vi "coag model selector.vi"(10 "scans":i32, 11 "Coagulant":T2={"flocculator volume (L)"=100.0, "clarifier volume (L)"=0.0, "dose updates per HRT"=0, "target clarified turbidity (NTU)"=0.3, "Coagulant mode"=enum."manual", "Coag dose [mg/L]"=0.0, "pump mL/rev"=0.0, "clarifier flow [L/s]"=0.5, "min Coag dose [mg/L]"=0.0, "max Coag dose [mg/L]"=0.0, "Steps"=3, "HRT response delay"=1, "Ku*"=1.0} {"HRT response delay" min=1 max=10 step=1; "Steps" min=3 step=1; "clarifier flow [L/s]" min=0.0001 max=1.0 step=0.0001; "target clarified turbidity (NTU)" min=0.1 max=5.0 step=0.01; "dose updates per HRT" min=1 max=100 step=1}) -> (7 "coag model":T1)   [LabVIEW 2019]
uses:
  coag.ctl
  model type.ctl
panel:
  # "min"
  # "max"
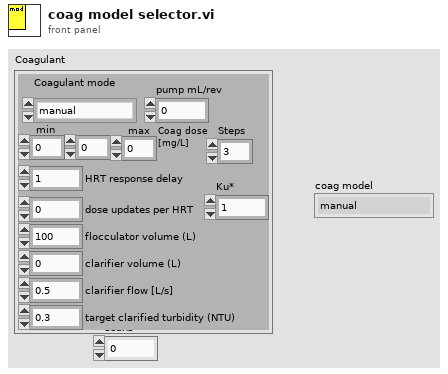
[diagram p1: front panel]
types:
  T1 = typedef "model type.ctl" = enum16{"manual", "ramp", "simple corrector", "linear regression"}
  T2 = typedef "coag.ctl" = cluster{"flocculator volume (L)":dbl, "clarifier volume (L)":dbl, "dose updates per HRT":u16, "target clarified turbidity (NTU)":dbl, "Coagulant mode":T1, "Coag dose [mg/L]":dbl, "pump mL/rev":dbl, "clarifier flow [L/s]":dbl, "min Coag dose [mg/L]":dbl, "max Coag dose [mg/L]":dbl, "Steps":u16, "HRT response delay":u32, "Ku*":dbl}
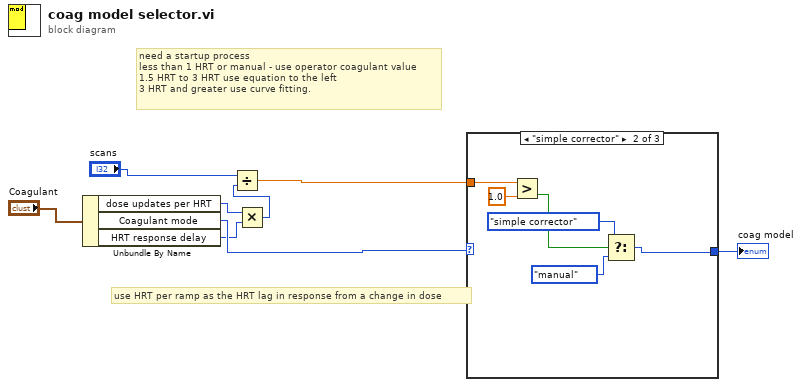
[diagram p0: block diagram]
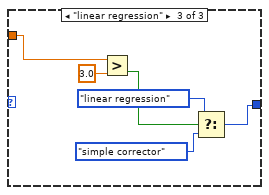
[diagram p3: hidden frame]
diagram:
  # "use HRT per ramp as the HRT lag in response from a change in dose"
  # "need a startup process \nless than 1 HRT or manual - use operator coagulant value\n1.5 HRT to 3 HRT use equation to the left\n3 HRT and greater use curve fitting."
  n1 = Unbundle By Name("Coagulant") -> ("dose updates per HRT"=w2:u16, "Coagulant mode"=w4:T1, "HRT response delay"=w3:u32)
  n2 = Multiply(x=w2, y=w3) -> (x*y=w1:u32)
  n3 = Divide(x="scans", y=w1) -> (x/y=w5:dbl)
  n4 = case shown="\"simple corrector\"" w4 {
    selector: w4 -> [w9 _ _]
    tunnel: [w9 w13 w16] -> w7
    tunnel: w5 -> [_ w12 w17]
    frame "manual", Default {
    }
    frame "simple corrector" {
      n5 = Greater?(x=w12, y=1.0) -> (0:w10:bool)
      n6 = Select(t=model_type."simple corrector" ("coag model"), s=w10, f=model_type."manual" ("coag model")) -> (s? t:f=w13:T1)
    }
    frame "linear regression" {
      n7 = Greater?(x=w17, y=3.0) -> (0:w18:bool)
      n8 = Select(t=model_type."linear regression" ("coag model"), s=w18, f=model_type."simple corrector" ("coag model")) -> (s? t:f=w16:T1)
    }
  }
  "coag model" <- w7
